vi "t3t.vi"(0 "T2":dbl, 1 "fuel (kg/s)":dbl, 2 "cpg":dbl, 3 "T3":dbl, 4 "cpa":dbl, 5 "Primery Air (kg/s)":dbl, 8 "Dilution Air (kg/s)":dbl) -> (7 "T03t":dbl)   [LabVIEW 2019]
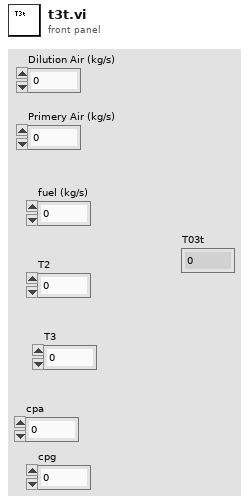
[diagram p1: front panel]
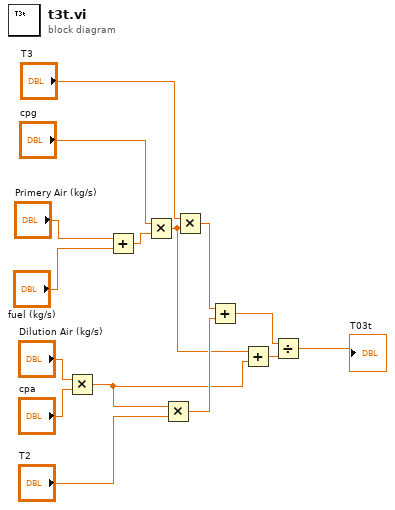
[diagram p0: block diagram]
diagram:
  n1 = Multiply(x="Dilution Air (kg/s)", y="cpa") -> (x*y=w1:dbl)
  n2 = Add(x="Primery Air (kg/s)", y="fuel (kg/s)") -> (x+y=w7:dbl)
  n3 = Multiply(x="cpg", y=w7) -> (x*y=w3:dbl)
  n4 = Multiply(x=w1, y="T2") -> (x*y=w8:dbl)
  n5 = Multiply(x="T3", y=w3) -> (x*y=w9:dbl)
  n6 = Add(x=w9, y=w8) -> (x+y=w5:dbl)
  n7 = Add(x=w3, y=w1) -> (x+y=w6:dbl)
  n8 = Divide(x=w5, y=w6) -> (x/y=→"T03t":dbl)
